vi "ChooseDuelist.vi"(10 "Id Manmarker":dbl format="%#_13g", 11 "IA State Input 2":T1={"our_robots"=[], "enemy_robots"=[], "balls"=[], "geometry"={"line_width"=0, "field_length"=0, "field_width"=0, "boundary_width"=0, "referee_width"=0, "goal_width"=0, "goal_depth"=0, "goal_wall_width"=0, "center_circle_radius"=0, "defense_radius"=0, "defense_stretch"=0, "free_kick_from_defense_dist"=0, "penalty_spot_from_field_line_dist"=0, "penalty_line_from_spot_dist"=0}, "IA Judge"={"stage"="", "command"="", "our_goalie_id"=0.0, "enemy_goalie_id"=0.0, "command enum"=enum."Halt", "Time"=enum."Azul"}, "Received Timestamp"=timestamp(0 s since 1904-01-01), "Events"={"Touch"=FALSE, "Ball out"=FALSE, "id touch"=0.0, "Ball out of \nVision"=FALSE, "Ball inside \nGoalie area"=FALSE, "Robot not responding"=FALSE, "Robots responding status"=[1.0, 1.0, 1.0, 1.0, 1.0, 1.0], "Enemy Ball \nPossession"=FALSE, "Pass State"=FALSE, "id end of pass"=0.0, "Kick"=FALSE, "Id ini Possession"=0.0, "Ball Possesion"=FALSE, "Id Possesion"=0.0}}) -> (2 "Defensores 2":u32[](array[numeric]), 3 "Id Duelist":u32)   [LabVIEW 2017]
uses:
  Core/AI Input.ctl
  Core/AI Robot.ctl
  Functions Enum.ctl
  AttackerStates.ctl
  Path Planning/RRT/PathDests.ctl
  Path Planning/RRT/PathDest.ctl
  Core/AI Ball.ctl
  Core/Field Size.ctl
  Core/AI Judge.ctl
  Command Enum.ctl
  Util/Events/Events.ctl
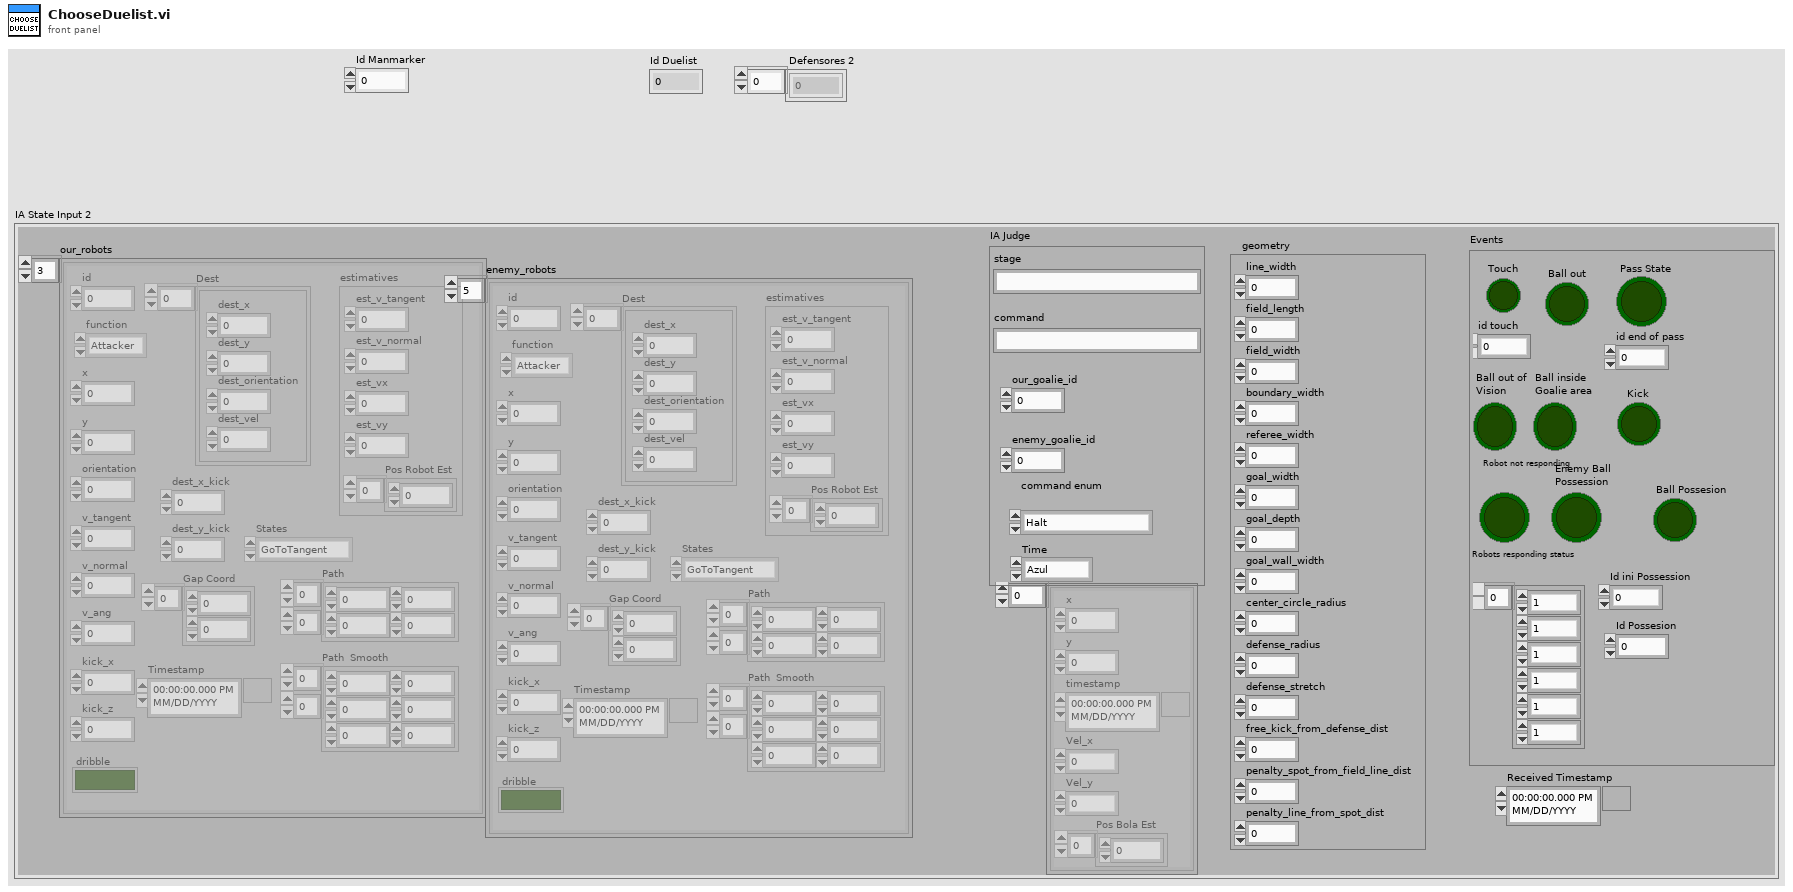
[diagram p1: front panel]
types:
  T1 = typedef "AI Input.ctl" = cluster{"our_robots":T2[], "enemy_robots":T2[], "balls":T7[], "geometry":T8, "IA Judge":T9, "Received Timestamp":timestamp, "Events":T11}
  T2 = typedef "AI Robot.ctl" = cluster{"id":u32, "function":T3, "x":dbl, "y":dbl, "orientation":dbl, "v_tangent":dbl, "v_normal":dbl, "v_ang":dbl, "kick_x":dbl, "kick_z":dbl, "dribble":bool, "Timestamp":timestamp, "estimatives":cluster{"est_v_tangent":dbl, "est_v_normal":dbl, "est_vx":dbl, "est_vy":dbl, "Pos Robot Est":dbl[]}, "dest_x_kick":dbl, "dest_y_kick":dbl, "Gap Coord":dbl[], "States":T4, "Path ":dbl[][], "Path  Smooth":dbl[][], "Dest":T5}
  T3 = typedef "Functions Enum.ctl" = enum16{"Attacker", "Goalie", "Defender", "Striker", "Goto 0", "Dummy", "Kicker", "ZigZag"}
  T4 = typedef "AttackerStates.ctl" = enum16{"Pass", "GoToTangent", "BallGetting", "GoToKick", ""}
  T5 = typedef "PathDests.ctl" = T6[]
  T6 = typedef "PathDest.ctl" = cluster{"dest_x":dbl, "dest_y":dbl, "dest_orientation":dbl, "dest_vel":dbl}
  T7 = typedef "AI Ball.ctl" = cluster{"x":dbl, "y":dbl, "timestamp":timestamp, "Vel_x":dbl, "Vel_y":dbl, "Pos Bola Est":dbl[]}
  T8 = typedef "Field Size.ctl" = cluster{"line_width":u32, "field_length":u32, "field_width":u32, "boundary_width":u32, "referee_width":u32, "goal_width":u32, "goal_depth":u32, "goal_wall_width":u32, "center_circle_radius":u32, "defense_radius":u32, "defense_stretch":u32, "free_kick_from_defense_dist":u32, "penalty_spot_from_field_line_dist":u32, "penalty_line_from_spot_dist":u32}
  T9 = typedef "AI Judge.ctl" = cluster{"stage":string, "command":string, "our_goalie_id":dbl, "enemy_goalie_id":dbl, "command enum":T10, "Time":enum16{"Azul", "Amarelo"}}
  T10 = typedef "Command Enum.ctl" = enum16{"Halt", "Stop", "Force Start", "PKA Normal Start", "Prepare Kickoff Ally", "PKE Normal Start", "Prepare Kickoff Enemy", "Prepare Penalty Ally", "PPA Normal Start", "Prepare Penalty Enemy", "PPE Normal Start", "Direct Free Enemy", "Direct Free Ally", "Indirect Free Enemy", "Indirect Free Ally", "Timeout Enemy", "Timeout Ally", "Goal Enemy", "Goal Ally", "Ball Placement Enemy", "Ball Placement Ally", "Normal Half Time", "Extra Time Break", "Extra Half Time", "None", "Post Game"}
  T11 = typedef "Events.ctl" = cluster{"Touch":bool, "Ball out":bool, "id touch":dbl, "Ball out of \nVision":bool, "Ball inside \nGoalie area":bool, "Robot not responding":bool, "Robots responding status":dbl[], "Enemy Ball \nPossession":bool, "Pass State":bool, "id end of pass":dbl, "Kick":bool, "Id ini Possession":dbl, "Ball Possesion":bool, "Id Possesion":dbl}
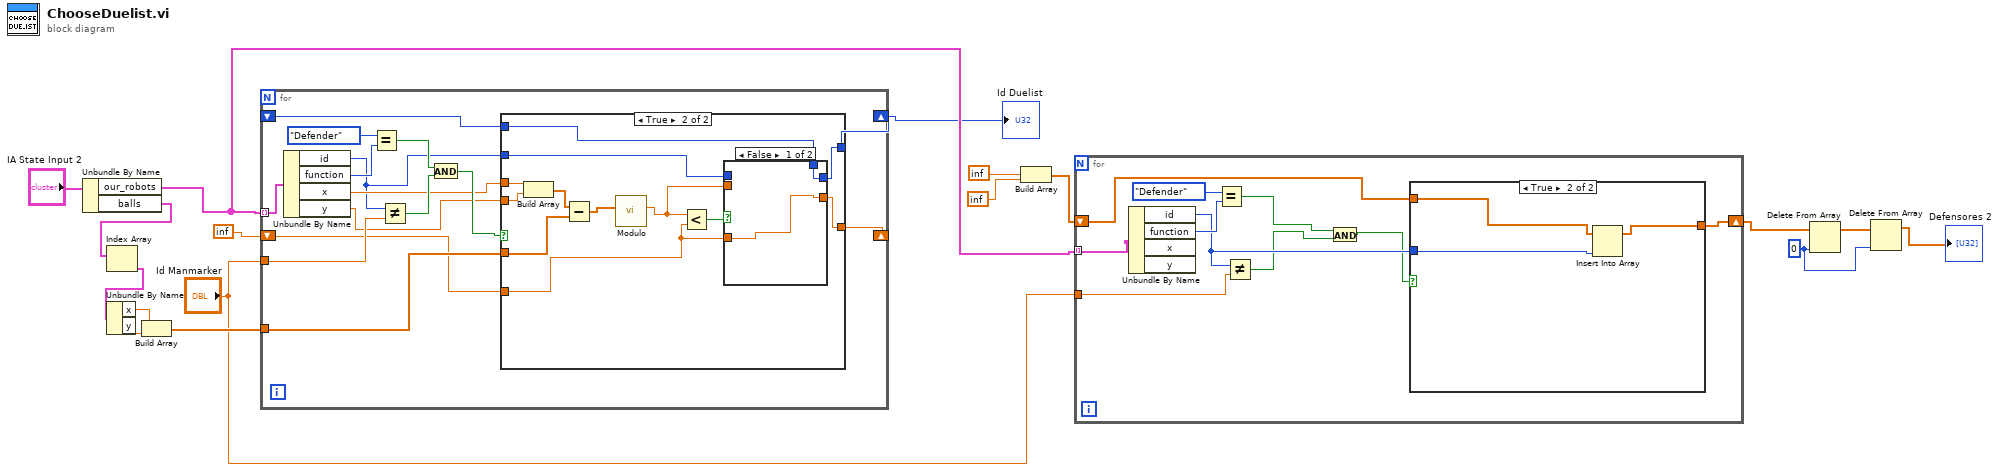
[diagram p0: block diagram]
diagram:
  w3 = 0 ("index")
  n1 = Unbundle By Name("IA State Input 2") -> ("our_robots"=w11:T2[], "balls"=w16:T7[])
  n2 = Index Array(array=w16) -> (element=w15:T7)  [unwired: 1 in]
  n3 = Unbundle By Name(w15) -> ("x"=w14:dbl, "y"=w13:dbl)
  n4 = Build Array(w14, w13) -> (w12:dbl[])
  n5 = for {
    tunnel: w11 -> [w32] mode=indexing
    tunnel: "Id Manmarker" -> [w28]
    tunnel: w12 -> [w23]
    shift-right: [w22] -> _
    shift-left: inf -> [w21]
    shift-right: [w20] -> w9
    shift-left: _ -> [w18]
    n6 = Unbundle By Name(w32) -> ("id"=w19:u32, "function"=w31:T3, "x"=w25:dbl, "y"=w24:dbl)
    n7 = Equal?(x=Functions_Enum."Defender", y=w31) -> (x = y?=w29:bool)
    n8 = Not Equal?(x=w19, y=w28) -> (x != y?=w27:bool)
    n9 = And(x=w29, y=w27) -> (x .and. y?=w26:bool)
    n10 = case shown="True" w26 {
      tunnel: w25 -> [_ w46]
      tunnel: w24 -> [_ w45]
      tunnel: w23 -> [_ w43]
      tunnel: [w33 w40] -> w22
      tunnel: w21 -> [w33 w35]
      tunnel: [w34 w38] -> w20
      tunnel: w19 -> [_ w37]
      tunnel: w18 -> [w34 w36]
      frame False {
      }
      frame True {
        n11 = Build Array(w46, w45) -> (w44:dbl[])
        n12 = Subtract(x=w44, y=w43) -> (x-y=w42:dbl[])
        n13 = call "Modulo.vi"("2D vector"=w42) -> ("Modulo"=w39:dbl)  [unwired: 10 in]
        n14 = Less?(x=w39, y=w35) -> (x < y?=w41:bool)
        n15 = case shown="False" w41 {
          tunnel: [w47 w50] -> w40
          tunnel: w39 -> [_ w50]
          tunnel: [w48 w49] -> w38
          tunnel: w37 -> [_ w49]
          tunnel: w36 -> [w48 _]
          tunnel: w35 -> [w47 _]
          frame False {
          }
          frame True {
          }
        }
      }
    }
  }
  "Id Duelist" <- w9
  n16 = Build Array(inf, inf) -> (w1:dbl[])
  n17 = for {
    tunnel: w11 -> [w58] mode=indexing
    tunnel: "Id Manmarker" -> [w57]
    shift-right: [w55] -> w6
    shift-left: w1 -> [w54]
    n18 = Unbundle By Name(w58) -> ("id"=w56:u32, "function"=w60:T3)  [unwired: 2 out]
    n19 = Equal?(x=Functions_Enum."Defender", y=w60) -> (x = y?=w53:bool)
    n20 = Not Equal?(x=w56, y=w57) -> (x != y?=w52:bool)
    n21 = And(x=w53, y=w52) -> (x .and. y?=w51:bool)
    n22 = case shown="True" w51 {
      tunnel: w56 -> [_ w64]
      tunnel: [w61 w63] -> w55
      tunnel: w54 -> [w61 w62]
      frame False {
      }
      frame True {
        n23 = Insert Into Array(array=w62, new element=w64) -> (w63:dbl[])  [unwired: 1 in]
      }
    }
  }
  n24 = Delete From Array(array=w6, index=w3) -> (array with subset deleted=w4:dbl[])  [unwired: 1 in, 1 out]
  n25 = Delete From Array(array=w4, index=w3) -> (array with subset deleted=→"Defensores 2":dbl[])  [unwired: 1 in, 1 out]
